vi "cameras_test.vi"() -> ()   [LabVIEW 2022 SP3]
doc: "Use this template to build a user interface event handler design pattern. Use this pattern for dialog boxes and other user interfaces. You also can create and execute user-defined events that the VI can handle the same way as user interface events."
uses:
  camera.ctl
  camera driver.ctl
  Vision.lvlib
panel:
  in  "Save Config":bool
  out "Image":T1(plugin-control)
  in  "End Stream":bool
  in  "Start Stream":bool
  in  "Snap Image":bool
  out "Available cameras":T2[](array[typedef])
  in  "Scan Cameras":bool
  in  "stop":bool
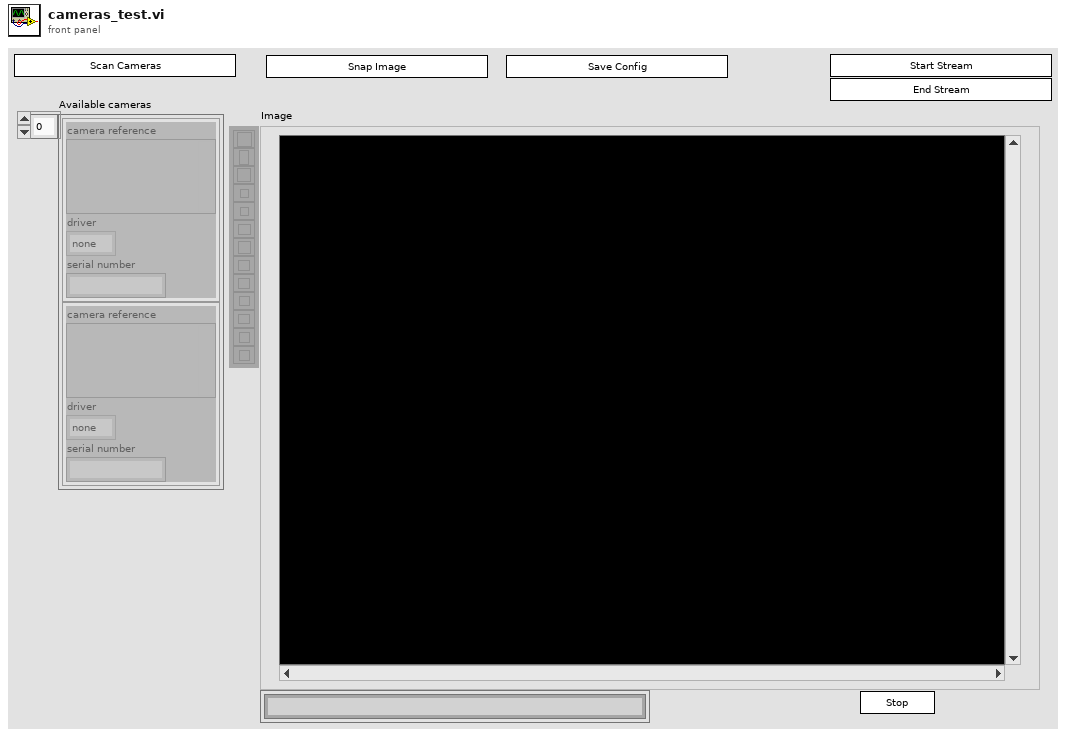
[diagram p1: front panel]
types:
  T1 = typedef "IMAQ Image.ctl" = refnum<image>
  T2 = typedef "Vision.lvlib/camera.ctl" = cluster{"camera reference":variant, "driver":T3, "serial number":string}
  T3 = typedef "Vision.lvlib/camera driver.ctl" = enum16{"none", "ueye"}
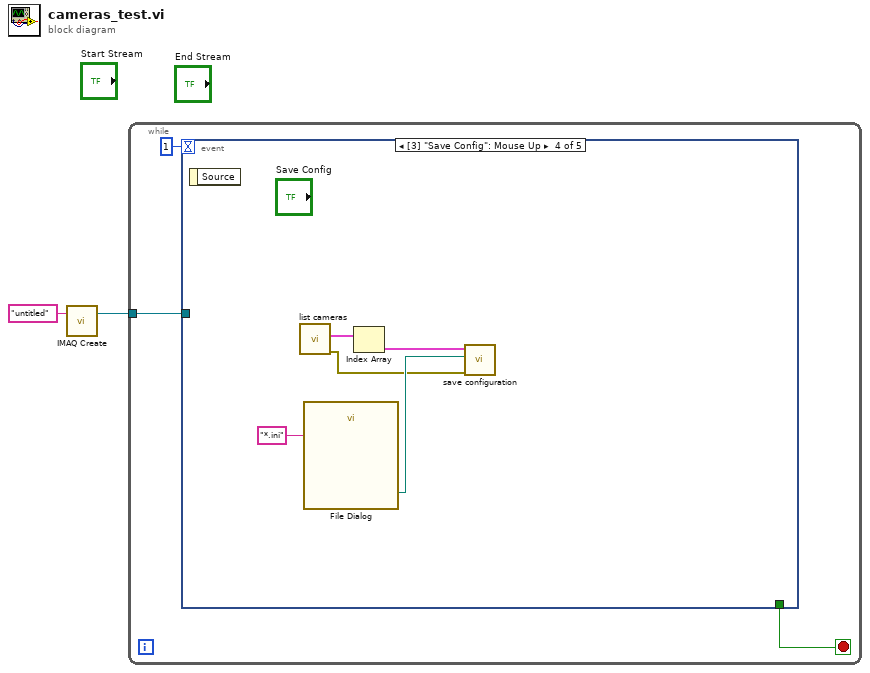
[diagram p0: block diagram]
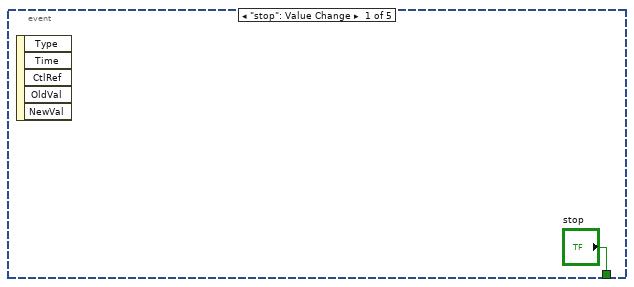
[diagram p2: hidden frame]
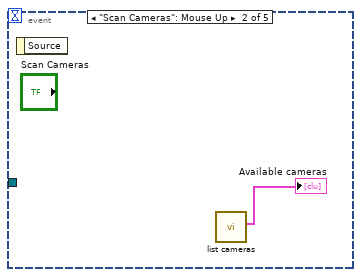
[diagram p3: hidden frame]
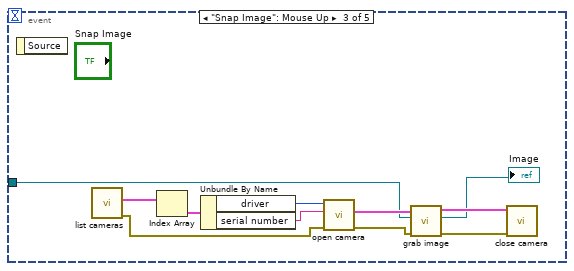
[diagram p4: hidden frame]
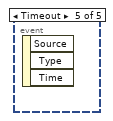
[diagram p5: hidden frame]
diagram:
  n1 = call "IMAQ Create"("Image Name"="untitled") -> ("New Image"=w1:T1)  [unwired: 4 in, 1 out]
  n2 = while {
    tunnel: w1 -> [w3]
    stop <- w5 stop-if-true
    n3 = event shown="[3] \"Save Config\": Mouse Up" {
      selector: _ -> [_ _ _ _ _]
      dyn-events: _ -> [_ _ _ _ _]
      timeout: 1 -> [_ _ _ _ _]
      tunnel: ["stop" _ _ _ _] -> w5
      tunnel: w3 -> [_ _ w8 _ _]
      event "stop": Value Change {
        n4 = event-data() -> ()  [unwired: 1 in, 5 out]
      }
      event "Scan Cameras": Mouse Up {
        n5 = event-data() -> ()  [unwired: 1 in, 1 out]
        n6 = call "list cameras.vi"() -> ("Cameras"=→"Available cameras":T2[])  [unwired: 10 in, 1 out]
      }
      event "Snap Image": Mouse Up {
        n7 = event-data() -> ()  [unwired: 1 in, 1 out]
        n8 = call "list cameras.vi"() -> ("error out"=w14:errorcluster, "Cameras"=w18:T2[])  [unwired: 10 in]
        n9 = Index Array(array=w18) -> (element=w17:T2)  [unwired: 1 in]
        n10 = Unbundle By Name(w17) -> ("driver"=w15:T3, "serial number"=w16:string)
        n11 = call "open camera.vi"("error in (no error)"=w14, "serial number"=w16, "driver"=w15) -> ("error out"=w12:errorcluster, "Camera"=w13:T2)  [unwired: 7 in]
        n12 = call "grab image.vi"("error in (no error)"=w12, "Image In"=w8, "Camera"=w13) -> ("error out"=w10:errorcluster, "Image Out"=→"Image":T1, "Camera out"=w11:T2)  [unwired: 6 in]
        n13 = call "close camera.vi"("error in (no error)"=w10, "Camera"=w11) -> ()  [unwired: 8 in, 2 out]
      }
      event "Save Config": Mouse Up {
        n14 = event-data() -> ()  [unwired: 1 in, 1 out]
        n15 = call "list cameras.vi"() -> ("error out"=w20:errorcluster, "Cameras"=w23:T2[])  [unwired: 10 in]
        n16 = call "File Dialog"("pattern (all files)"="*.ini" ("pattern label")) -> ("selected path"=w21:path)  [unwired: 11 in, 3 out]
        n17 = Index Array(array=w23) -> (element=w22:T2)  [unwired: 1 in]
        n18 = call "save configuration.vi"("error in (no error)"=w20, "Path"=w21, "Camera"=w22) -> ()  [unwired: 7 in, 2 out]
      }
      event Timeout {
        n19 = event-data() -> ()  [unwired: 1 in, 3 out]
      }
    }
  }
